vi "xt.vi"(10 "stages":T2[](array[typedef]) {"t (s)" format="%#_6e"; "v_i (m/s)" format="%#_6e"; "a (m / s^2)" format="%#_6e"; "d (m)" format="%#_6e"; "v_f (m/s)" format="%#_6e"}, 11 "dt (s)":dbl=1e-08 format="%#_6p") -> (1 "XT":cluster{"time":dbl[], "velocity":dbl[]}[](array[cluster]), 2 "output":T1, 3 "num_steps":i32)   [LabVIEW 2013, in "wf_tools.lvlib"]
uses:
  wf_tools.lvlib
  stage.ctl
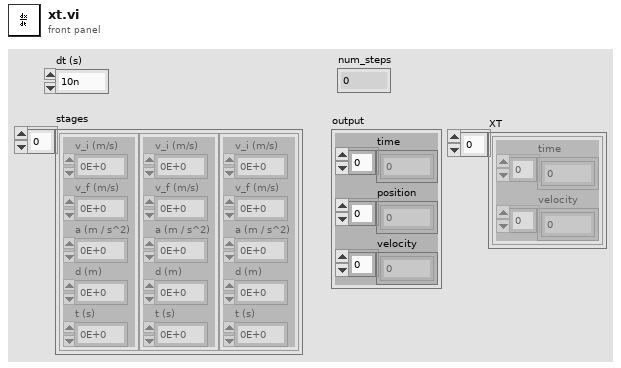
[diagram p1: front panel]
types:
  T1 = cluster{"time":dbl[], "position":dbl[], "velocity":dbl[]}
  T2 = typedef "wf_tools.lvlib/stage.ctl" = cluster{"v_i (m/s)":dbl, "v_f (m/s)":dbl, "a (m / s^2)":dbl, "d (m)":dbl, "t (s)":dbl}
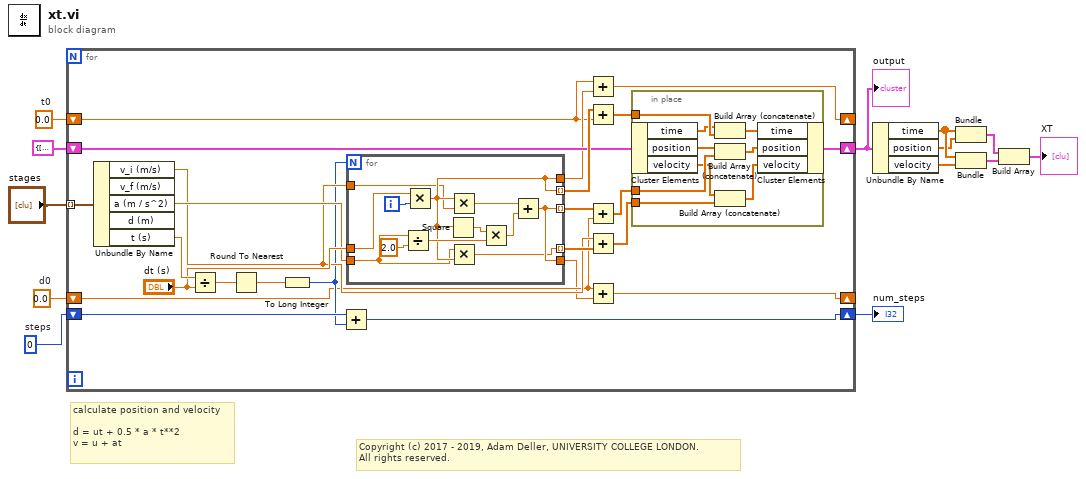
[diagram p0: block diagram]
diagram:
  w9 = 0  # steps
  w11 = 0.0  # d0
  w13 = 0.0  # t0
  # "Copyright (c) 2017 - 2019, Adam Deller, UNIVERSITY COLLEGE LONDON.\nAll rights reserved."
  # "calculate position and velocity\n\nd = ut + 0.5 * a * t**2\nv = u + at"
  n1 = for {
    shift-right: [w18] -> _
    shift-left: w13 -> [w17]
    tunnel: "stages" -> [w37] mode=indexing
    shift-right: [w14] -> _
    shift-left: w11 -> [w16]
    shift-right: [w24] -> w7
    shift-left: T1 {"time"=[], "position"=[], "velocity"=[]} ("trap") -> [w25]
    shift-right: [w20] -> w8
    shift-left: w9 -> [w22]
    n2 = Unbundle By Name(w37) -> ("v_i (m/s)"=w23:dbl, "a (m / s^2)"=w32:dbl, "t (s)"=w36:dbl)  [unwired: 2 out]
    n3 = Divide(x=w36, y="dt (s)") -> (x/y=w35:dbl)
    n4 = Round To Nearest(number=w35) -> (nearest integer value=w34:dbl)
    n5 = To Long Integer(number=w34) -> (32bit integer=w21:i32)
    n6 = Add(x=w22, y=w21) -> (x+y=w20:i32)
    n7 = for {
      N: w21 -> [_]
      tunnel: [w51] -> w30 mode=indexing
      tunnel: [w50] -> w31 mode=indexing
      tunnel: "dt (s)" -> [w52]
      tunnel: w32 -> [w49]
      tunnel: [w51] -> w15
      tunnel: [w50] -> w19
      tunnel: [w48] -> w28 mode=indexing
      tunnel: w23 -> [w47]
      i -> [w58]
      n8 = Divide(x=w49, y=2.0) -> (x/y=w55:dbl)
      n9 = Multiply(x=w52, y=w58) -> (x*y=w50:dbl)
      n10 = Square(x=w50) -> (x^2=w54:dbl)
      n11 = Multiply(x=w50, y=w47) -> (x*y=w56:dbl)
      n12 = Multiply(x=w49, y=w50) -> (x*y=w48:dbl)
      n13 = Multiply(x=w54, y=w55) -> (x*y=w53:dbl)
      n14 = Add(x=w56, y=w53) -> (x+y=w51:dbl)
    }
    n15 = Add(x=w17, y=w19) -> (x+y=w18:dbl)
    n16 = Add(x=w31, y=w17) -> (x+y=w27:dbl[])
    n17 = Add(x=w30, y=w16) -> (x+y=w29:dbl[])
    n18 = Add(x=w23, y=w28) -> (x+y=w26:dbl[])
    n19 = Add(x=w16, y=w15) -> (x+y=w14:dbl)
    n20 = in-place {
      in-place-border: w29 -> [w46]
      in-place-border: w27 -> [w45]
      in-place-border: w26 -> [w44]
      n21 = in-place-cluster #1(w25) -> ("time"=w43:dbl[], "position"=w41:dbl[], "velocity"=w39:dbl[])
      n22 = Build Array (concatenate)(w43, w45) -> (w42:dbl[])
      n23 = Build Array (concatenate)(w41, w46) -> (w40:dbl[])
      n24 = Build Array (concatenate)(w39, w44) -> (w38:dbl[])
      n25 = in-place-cluster #1("time"=w42, "position"=w40, "velocity"=w38) -> (w24:T1)
    }
  }
  "output" <- w7
  "num_steps" <- w8
  n26 = Unbundle By Name(w7) -> ("time"=w6:dbl[], "position"=w5:dbl[], "velocity"=w4:dbl[])
  n27 = Bundle("time"=w6, "position"=w5) -> (w2:cluster{"time":dbl[], "position":dbl[]})  [unwired: 1 in]
  n28 = Bundle("time"=w6, "velocity"=w4) -> (w3:cluster{"time":dbl[], "velocity":dbl[]})  [unwired: 1 in]
  n29 = Build Array(w2, w3) -> (→"XT":cluster{"time":dbl[], "velocity":dbl[]}[])
